vi "Ack needed.vi"(11 "IPublish in":refnum<class "IPublish.lvclass">) -> (2 "Ack needed?":bool, 3 "IPublish out":refnum<class "IPublish.lvclass">)   [LabVIEW 2020, in "wamplv.lvlib" / "IPublish.lvclass"]
uses:
  IPublish.lvclass
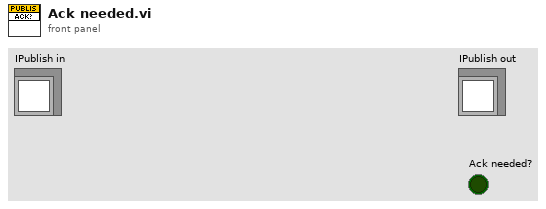
[diagram p1: front panel]
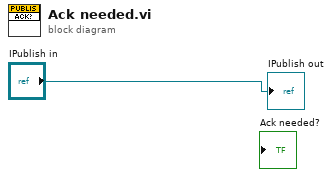
[diagram p0: block diagram]
diagram:
  "IPublish out" <- "IPublish in"
